vi "CAN Rx Judge.vi"(11 "data":u8[](array[numeric]) format="%.0x") -> (3 "result":bool, 5 "empty?":bool)   [LabVIEW 2024]
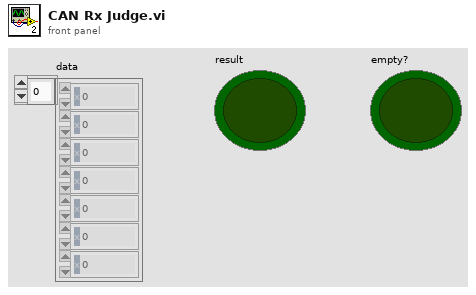
[diagram p1: front panel]
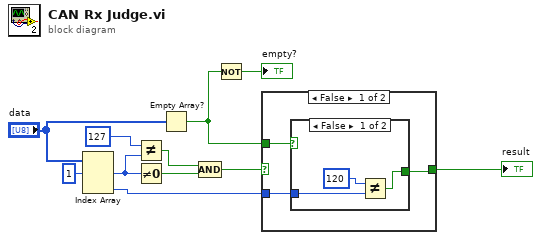
[diagram p0: block diagram]
diagram:
  n1 = Index Array(array="data", index #1=1 ("索引")) -> (element #1=w8:u8, element #3=w4:u8)  [unwired: 2 in, 1 out]
  n2 = Not Equal?(x=u8 127, y=w8) -> (x != y?=w7:bool)
  n3 = Not Equal To 0?(x=w8) -> (x != 0?=w10:bool)
  n4 = Empty Array?(array="data") -> (empty?=w2:bool)
  n5 = Compound Arithmetic op=AND ("复合运算")(w7, w10) -> (w6:bool)
  n6 = Not(x=w2) -> (.not. x?=→"empty?":bool)
  n7 = case shown="False" w6 {
    selector: w6 -> [_ w18]
    tunnel: [w13 w18] -> w5
    tunnel: w4 -> [w14 _]
    tunnel: w2 -> [w12 _]
    frame False {
      n8 = case shown="False" w12 {
        tunnel: w14 -> [w17 _]
        tunnel: [w15 _] -> w13
        frame False {
          n9 = Not Equal?(x=u8 120, y=w17) -> (x != y?=w15:bool)
        }
        frame True {
        }
      }
    }
    frame True {
    }
  }
  "result" <- w5
